vi "Read Dips.vi"(8 "error in":errorcluster, 10 "Default":i32, 11 "HBDevRef":T1) -> (0 "error out":errorcluster)   [LabVIEW 2016, in "Huskie Swerve.lvlib"]
uses:
  Huskie Swerve.lvlib
  <vilib>/Rock Robotics/WPI/SerialPort/WPI_SerialPortRef.ctl
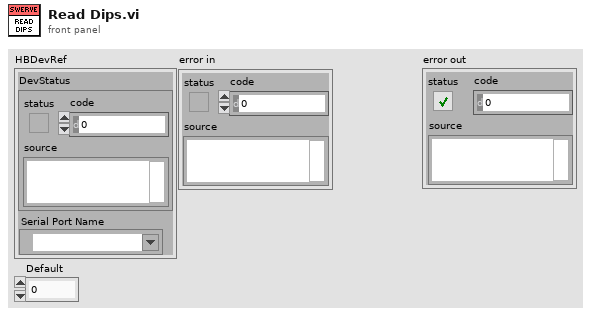
[diagram p1: front panel]
types:
  T1 = typedef "WPI_SerialPortRef.ctl" = cluster{"DevStatus":errorcluster, "Serial Port Name":refnum<visa-resource-name>}
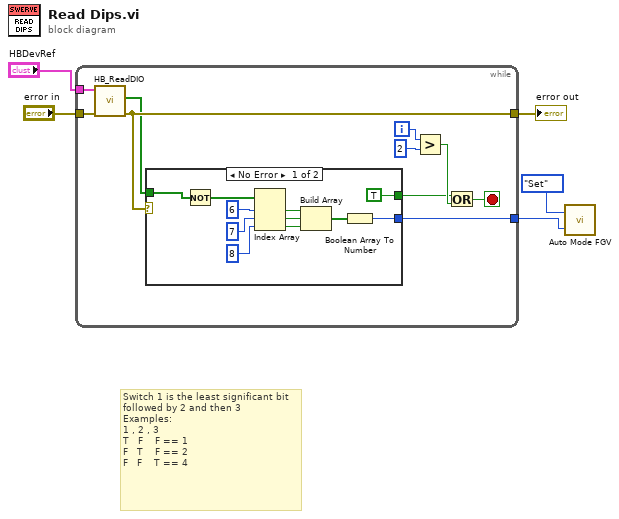
[diagram p0: block diagram]
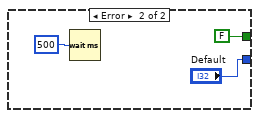
[diagram p2: hidden frame]
diagram:
  # "Switch 1 is the least significant bit\nfollowed by 2 and then 3\nExamples:\n1 , 2 , 3\nT   F    F == 1\nF   T    F == 2\nF   F    T == 4"
  n1 = while {
    tunnel: "HBDevRef" -> [w15]
    tunnel: [w6] -> w1
    tunnel: "error in" -> [w14]
    tunnel: [w13] -> w3
    i -> [w12]
    stop <- w8 stop-if-true
    n2 = call <vilib>:"HB_ReadDIO.vi"("error in (no error)"=w14, "HBDeviceRef"=w15) -> ("error out"=w13:errorcluster, "All Digital Input Vals"=w7:bool[])  [unwired: 7 in, 1 out]
    n3 = case shown="No Error" w13 {
      tunnel: [TRUE FALSE] -> w9
      tunnel: w7 -> [w17 _]
      tunnel: [w16 "Default"] -> w6
      frame No Error {
        n4 = Not(x=w17) -> (.not. x?=w22:bool[])
        n5 = Index Array(array=w22, index #1=6 ("index"), index #2=7 ("index"), index #3=8 ("index")) -> (element #1=w21:bool, element #2=w20:bool, element #3=w19:bool)
        n6 = Build Array(w21, w20, w19) -> (w18:bool[])
        n7 = Boolean Array To Number(Boolean array=w18) -> (number=w16:u32)
      }
      frame Error {
        n8 = Wait (ms)(milliseconds to wait=u32 500) -> ()  [unwired: 1 out]
      }
    }
    n9 = Greater?(x=w12, y=2) -> (0:w10:bool)
    n10 = Or(x=w9, y=w10) -> (x .or. y?=w8:bool)
  }
  "error out" <- w3
  n11 = call "Auto Mode FGV.vi"("New Auto Mode"=w1, "Action"=enum16{"Set", "Get"}."Set") -> ()  [unwired: 1 out]
